vi "Read Attributes Found.vi"(8 "error in (no error)":errorcluster, 11 "CS++BaseActor in":refnum<class "CS++BaseActor.lvclass">) -> (0 "error out":errorcluster, 2 "Attributes Found":bool, 3 "CS++BaseActor out":refnum<class "CS++BaseActor.lvclass">)   [LabVIEW 2013, in "CS++BaseActor.lvlib" / "CS++BaseActor.lvclass"]
uses:
  CS++BaseActor.lvclass
  CS++BaseActor.lvclass/CS++BaseActor.ctl
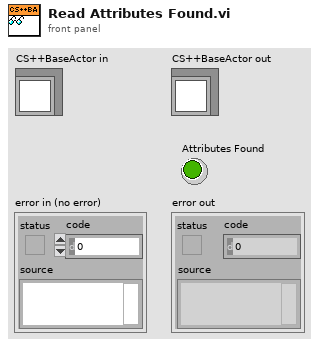
[diagram p1: front panel]
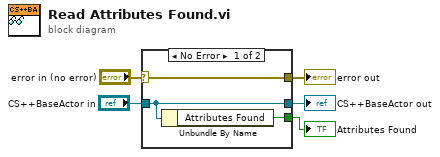
[diagram p0: block diagram]
diagram:
  n1 = case shown="No Error" "error in (no error)" {
    selector: "error in (no error)" -> [w8 w9]
    tunnel: [w8 w9] -> w4
    tunnel: [w7 w10] -> w2
    tunnel: "CS++BaseActor in" -> [w7 w10]
    tunnel: [w6 _] -> w1
    frame No Error {
      n2 = Unbundle By Name(w7) -> ("Attributes Found"=w6:bool)
    }
    frame Error {
    }
  }
  "error out" <- w4
  "CS++BaseActor out" <- w2
  "Attributes Found" <- w1
